vi "AIT 1553 - Create BC Sysdef Tree Acyclic Frames.vi"(8 "error in":errorcluster, 10 "Section Ptr":T1 format="%.0x", 11 "Acyclic_Frames":T2[](array[typedef])) -> (0 "error out":errorcluster, 2 "Section Ptr Out":T1 format="%.0x")   [LabVIEW 2011]
uses:
  <vilib>/NI Veristand/Custom Device API/Custom Device Item Ref.ctl
  Controls/1553_Acyclic_Frame.ctl
  <vilib>/NI Veristand/Custom Device API/Custom Device Channel.ctl
  <vilib>/NI Veristand/Custom Device API/Custom Device Channel Type.ctl
  Controls and Global/Global.vi
  <vilib>/NI Veristand/Custom Device API/Custom Device API.lvlib
  AIT 1553 Custom Device.lvlib
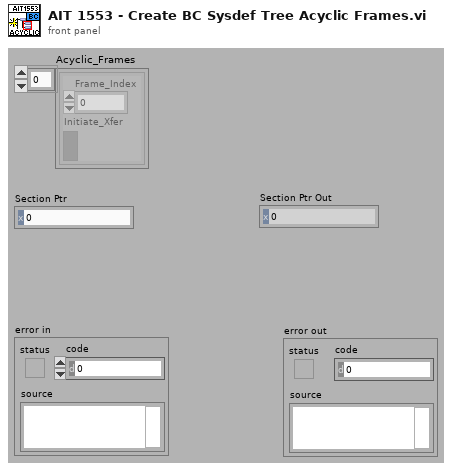
[diagram p1: front panel]
types:
  T1 = typedef "Custom Device API.lvlib/Custom Device Item Ref.ctl" = u64
  T2 = typedef "AIT 1553 Custom Device.lvlib/1553_Acyclic_Frame.ctl" = cluster{"Frame_Index":u8, "Initiate_Xfer":bool}
  T3 = typedef "Custom Device API.lvlib/Custom Device Channel.ctl" = cluster{"Type":T4, "Units":string, "Default Value":dbl, "Faultable":bool, "Scalable":bool}
  T4 = typedef "Custom Device API.lvlib/Custom Device Channel Type.ctl" = enum16{"Input", "Output"}
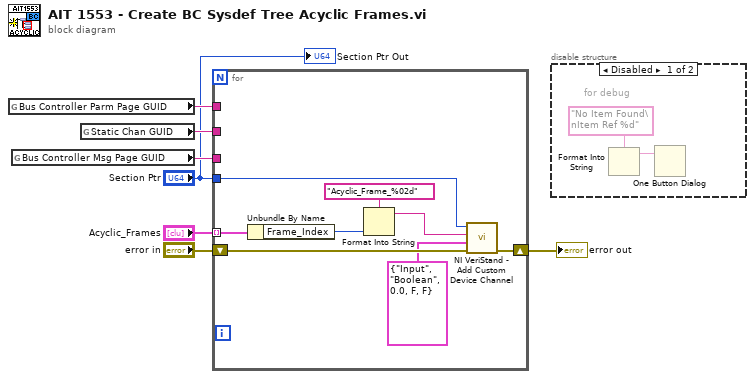
[diagram p0: block diagram]
diagram:
  n1 = global read "Global.vi" "Bus Controller Parm Page GUID"() -> (w3:string)
  n2 = global read "Global.vi" "Bus Controller Msg Page GUID"() -> (w5:string)
  n3 = global read "Global.vi" "Static Chan GUID"() -> (w4:string)
  n4 = for {
    shift-right: [w8] -> w7
    shift-left: "error in" -> [w15]
    tunnel: "Section Ptr" -> [w12]
    tunnel: "Acyclic_Frames" -> [w11] mode=indexing
    tunnel: w5 -> [_]
    tunnel: w4 -> [_]
    tunnel: w3 -> [_]
    n5 = Unbundle By Name(w11) -> ("Frame_Index"=w10:u8)
    n6 = Format Into String(format string="Acyclic_Frame_%02d" ("Channel Name"), w10) -> (resulting string=w9:string)  [unwired: 2 in, 1 out]
    n7 = call <vilib>:"NI VeriStand - Add Custom Device Channel.vi"("error in (no error)"=w15, "Channel"=T3 {"Type"=enum."Input", "Units"="Boolean", "Default Value"=0.0, "Faultable"=FALSE, "Scalable"=FALSE}, "Channel Name"=w9, "Parent Ref in"=w12) -> ("error out"=w8:errorcluster)  [unwired: 4 in, 3 out]
  }
  "error out" <- w7
  n8 = disable-structure shown="Disabled" {
    frame Disabled {
      # "for debug"
      n9 = Format Into String(format string="No Item Found\nItem Ref %d" ("message")) -> (resulting string=w18:string, w16:T1)  [unwired: 2 in, 1 out]
      n10 = One Button Dialog(message=w18) -> (true=w19:bool)  [unwired: 1 in]
    }
    frame Enabled {
    }
  }
  "Section Ptr Out" <- "Section Ptr"
